vi "From string.vi"(8 "error in (no error)":errorcluster, 10 "String":string, 11 "Power control in":refnum<class "Power control.lvclass">) -> (0 "error out":errorcluster, 3 "Power control out":refnum<class "Power control.lvclass">)   [LabVIEW 2015, in "Power control.lvclass"]
uses:
  Power control.lvclass
  Power control.lvclass/Power control.ctl
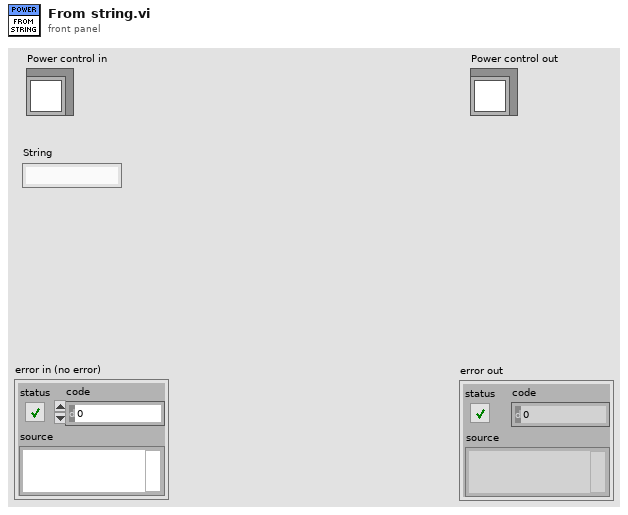
[diagram p1: front panel]
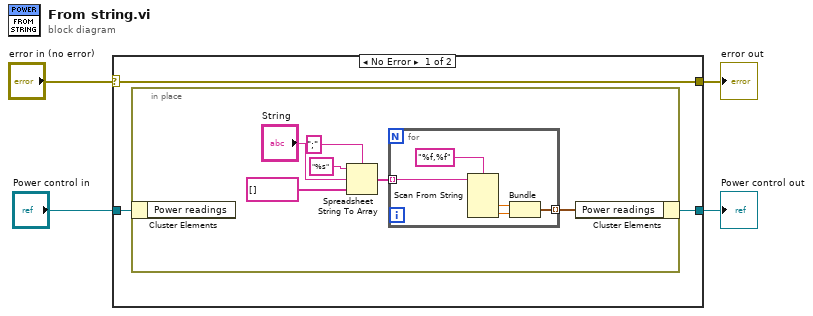
[diagram p0: block diagram]
diagram:
  n1 = case shown="No Error" "error in (no error)" {
    selector: "error in (no error)" -> [w5 w20]
    tunnel: "Power control in" -> [w7 w19]
    tunnel: [w6 w19] -> w3
    tunnel: [w5 w20] -> w1
    frame No Error {
      n2 = in-place {
        n3 = in-place-cluster #1(w7) -> ()  [unwired: 1 out]
        n4 = Spreadsheet String To Array(delimiter (Tab)=";", format string="%s", spreadsheet string="String", array type (2D Dbl)=string[] []) -> (array=w9:string[])
        n5 = for {
          tunnel: w9 -> [w17] mode=indexing
          tunnel: [w14] -> w8 mode=indexing
          n6 = Scan From String(format string="%f,%f", input string=w17) -> (output 1=w16:dbl, output 2=w15:dbl)  [unwired: 4 in, 3 out]
          n7 = Bundle(w16, w15) -> (w14:cluster{dbl, dbl})  [unwired: 1 in]
        }
        n8 = in-place-cluster #1("Power readings"=w8) -> (w6:refnum<class "Power control.lvclass">)
      }
    }
    frame Error {
    }
  }
  "Power control out" <- w3
  "error out" <- w1
